vi "Save single image with metadata to Tiff file.vi"(6 "ImageDescription string\n(must be at least 5 char long if used)":string=" Four score and seven years ago our fathers brought forth on this continent, a new nation, conceived in Liberty, and dedicated to the proposition that all men are created equal.\n\nNow we are engaged in a great civil war, testing whether that nation, or any nation so conceived and so dedicated, can long endure. We are met on a great battle-field of that war. We have come to dedicate a portion of that field, as a final resting place for those who here gave their lives that that nation might live. It is altogether fitting and proper that we should do this.\n\nBut, in a larger sense, we can not dedicate -- we can not consecrate -- we can not hallow -- this ground. The brave men, living and dead, who struggled here, have consecrated it, far above our poor power to add or detract. The world will little note, nor long remember what we say here, but it can never forget what they did here. It is for us the living, rather, to be dedicated here to the unfinished work which they who fought here have thus far so nobly advanced. It is rather for us to be here dedicated to the great task remaining before us -- that from these honored dead we take increased devotion to that cause for which they gave the last full measure of devotion -- that we here highly resolve that these dead shall not have died in vain -- that this nation, under God, shall have a new birth of freedom -- and that government of the people, by the people, for the people, shall not perish from the earth. ", 8 "error in":errorcluster, 9 "Compression Type (None)":i32(ring) items=["None", "JPEG", "Run Length Encoded", "Zip"], 10 "file":path, 11 "Img (U8, I16, U16)":T1) -> (0 "error out":errorcluster, 3 "Image Out (duplicate)":T1)   [LabVIEW 2013, in "Tiff reader.lvlib"]
doc: "This .vi saves an image to a tiff file specified and adds the \"Custom Data\" strings attached to the images to the Tiff file metadata."
uses:
  Tiff reader.lvlib
  <vilib>/vision/Image Controls.llb/IMAQ Image.ctl
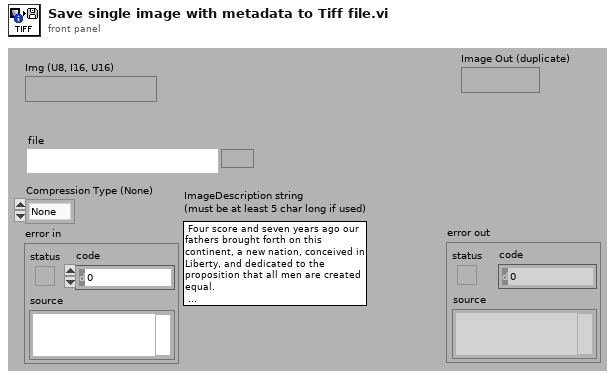
[diagram p1: front panel]
types:
  T1 = typedef "IMAQ Image.ctl" = refnum<image>
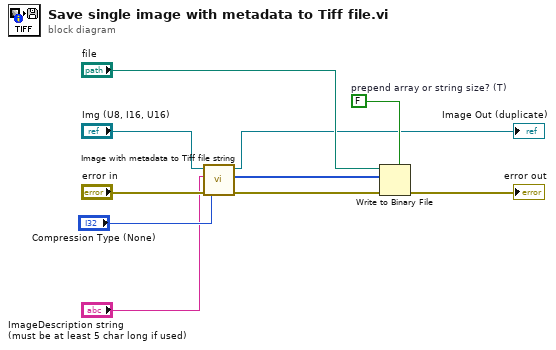
[diagram p0: block diagram]
diagram:
  w9 = FALSE  # prepend array or string size? (T)
  n1 = call "Image with metadata to Tiff file string.vi"("error in"="error in", "Compression Type (None)"="Compression Type (None)", "ImageDescription string\n(must be at least 5 char long)"="ImageDescription string\n(must be at least 5 char long if used)", "img"="Img (U8, I16, U16)") -> ("error out"=w4:errorcluster, "Tiff file out (unsigned byte array)"=w10:u8[], "Image Out (duplicate)"=→"Image Out (duplicate)":T1)  [unwired: 1 out]
  n2 = Write to Binary File(file (use dialog)="file", data=w10, error in=w4, 5:w9) -> (error out=→"error out":errorcluster)  [unwired: 4 out]
